vi "Multi-Device Tx Streaming Time (Host).vi"() -> ()   [LabVIEW 2015]
doc: "This template is for the Simple NI-USRP Streaming design, a design that shows the basics of streaming data to and from an NI USRP-294x/295x device. Refer to the block diagram for more information about how to use this template."
uses:
  <vilib>/Utility/error.llb/DialogType.ctl
  <vilib>/userdefined/Silver/nirio_resource_slv.ctl
  SubVIs/Start Trigger.ctl
panel:
  in  "config tab":enum32{"Tx Configuration"}(tab)
  in  "tx config":T2={"rf enable 0"=TRUE, "rf config 0"={"antenna"="TX1", "frequency"=2000000000.0, "lo frequency"=-1.0, "level"=0.0}, "rf enable 1"=TRUE, "rf config 1"={"antenna"="TX1", "frequency"=2000000000.0, "lo frequency"=-1.0, "level"=0.0}, "transfer mode"=enum."Finite", "sample rate"=10000000.0, "number of samples"=8192, "start trigger"=enum."Future Time Event", "tone frequency"=100000.0} {"tone frequency" format="%#.3pHz"; "sample rate" format="%#.3pS/s"; "rf config 0"."level" format="%#_gdBm"; "rf config 0"."lo frequency" format="%#.3pHz"; "rf config 0"."frequency" format="%#.3pHz"; "rf config 1"."level" format="%#_gdBm"; "rf config 1"."lo frequency" format="%#.3pHz"; "rf config 1"."frequency" format="%#.3pHz"}
  in  "tx.stop":bool
  out "generating":bool caption="Generating"
  in  "USRP RIO devices":T3[](array[typedef])=["RIO0", "RIO1"] caption="USRP RIO Devices"
  in  "reference frequency source":string(combo)="REF IN" caption="Reference Frequency Source"
  in  "indicator tab":T4(tab)
  out "tx.waveform":waveform(dbl)[](graph) caption="Output Waveform"
  out "tx.coerced config":T5(array[cluster]) caption="Tx" {"coerced sample rates" format="%#.3pS/s"; "coerced levels" format="%#.3gdBm"; "coerced lo frequencies" format="%#.3pHz"; "coerced frequencies" format="%#.3pHz"}
  # "This template is for the Simple NI-USRP Streaming design, a design that shows the basics of streaming data on an NI 294x/295x device. See the block diagram for more information on how to use this template."
  # "Multi-Device Tx Streaming with Time"
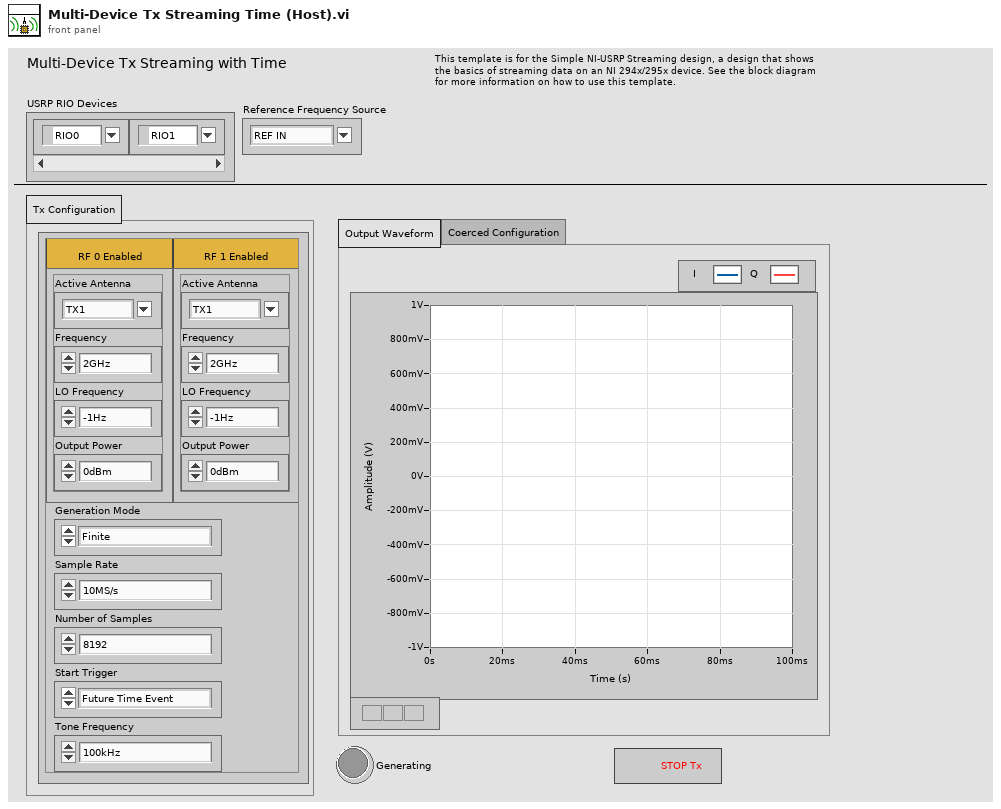
[diagram p1: front panel]
types:
  T1 = typedef "Start Trigger.ctl" = enum8{"Software", "Digital Edge", "Rx Start Trigger", "Tx Start Trigger", "Immediate", "Future Time Event"}
  T2 = cluster{"rf enable 0":bool, "rf config 0":cluster{"antenna":string, "frequency":dbl, "lo frequency":dbl, "level":dbl}, "rf enable 1":bool, "rf config 1":cluster{"antenna":string, "frequency":dbl, "lo frequency":dbl, "level":dbl}, "transfer mode":enum16{"Finite", "Continuous"}, "sample rate":dbl, "number of samples":u32, "start trigger":T1, "tone frequency":dbl}
  T3 = typedef "nirio_resource_slv.ctl" = tag
  T4 = enum32{"Output Waveform", "Coerced Configuration"}
  T5 = cluster{"coerced frequencies":dbl[], "coerced lo frequencies":dbl[], "coerced levels":dbl[], "coerced sample rates":dbl[]}[]
  T6 = typedef "DialogType.ctl" = u16
  T7 = cluster{"tx config":cluster{"rf enable 0":bool, "rf config 0":cluster{"antenna":string, "frequency":dbl, "lo frequency":dbl, "level":dbl}, "rf enable 1":bool, "rf config 1":cluster{"antenna":string, "frequency":dbl, "lo frequency":dbl, "level":dbl}, "transfer mode":enum16{"Finite", "Continuous"}, "sample rate":dbl, "number of samples":u32, "start trigger":T1, "tone frequency":dbl}, "reference frequency source":string, "tx.enabled channels":string[], "I":i16[], "Q":i16[], "tx.coerced configurations":cluster{"coerced frequencies":dbl[], "coerced lo frequencies":dbl[], "coerced levels":dbl[], "coerced sample rates":dbl[]}}
  T8 = typedef "niUsrpRio Config v1 Host.lvlib/niUsrpRio Session.ctl" = cluster{"FPGA Interface":refnum<k20>, "RIO Interface Number":u32, "Data Clock Rate":u32, "FPGA Data Clock Rate":u32, "Global Settings Register Bus":T9, "Radio 0 Settings Register Bus":T9, "Radio 1 Settings Register Bus":T9, "Radio Settings Bus Semaphore":T10, "DB Queues":T11[], "Characterization Data Valid?":bool, "EEPROM Header":T12, "Device Data Header":T13, "EEPROM Characterization Header":T14, "Characterization Data":T15[], "FPGA Current Version":u32, "FPGA Oldest Compatible Version":u32, "Fixed Logic Current Version":u32, "Fixed Logic Oldest Compatible Version":u32, "FPGA Radio Settings Bus Current Version":u32, "FPGA Radio Settings Bus Oldest Compatible Version":u32, "FPGA Board Config Current Version":u32, "FPGA Board Config Oldest Compatible Version":u32, "Daughterboard Clock Rate":u32}
  T9 = typedef "niInstr Register Bus v0 Host.lvlib/Register Bus Session.ctl" = refnum<queue>
  T10 = typedef "Semaphore RefNum" = refnum<k1>
  T11 = typedef "niUsrpRio Config v1 Host.lvlib/DB Queue Reference.ctl" = refnum<queue>
  T12 = typedef "niUsrpRio Config v1 Host.lvlib/EEPROM Header.ctl" = cluster{"Checksum":u32, "Product Code":u16, "Hardware Current Version":u16, "Hardware Oldest Compatible Version":u16, "EEPROM Map Current Version":u16, "EEPROM Map Oldest Compatible Version":u16, "User Password":string, "Pointer to Factory Header":u32, "Pointer to User Header":u32, "Recommended Interval":u16, "Number of Reserved Bytes":i32, "Number of Daughterboards":u8, "Daughterboard IDs":u16[], "Daughterboard Serial Numbers":string[]}
  T13 = typedef "niUsrpRio Config v1 Host.lvlib/EEPROM Device Data Header.ctl" = cluster{"Checksum":u32, "Number of Channels":u8, "Number of Gain Settings":u16[], "Pointer to Characterization Data":u32[], "Number of Reserved Bytes":i32, "Number of Frequencies":u16[]}
  T14 = typedef "niUsrpRio Config v1 Host.lvlib/EEPROM Characterization Header.ctl" = cluster{"Checksum":u32, "Date":timestamp, "Temperature":sgl, "Misc. Info":string, "Pointer to Device Data Header":u32, "Number of Reserved Bytes":i32}
  T15 = typedef "niUsrpRio Config v1 Host.lvlib/Characterization Data.ctl" = cluster{"Gains[dB]":dbl[], "Frequencies [Hz]":dbl[], "IQ Imbalance Table":T16[], "Measured Gains[dB]":dbl[][]}
  T16 = typedef "niUsrpRio Config v1 Host.lvlib/IQ Imbalance.ctl" = cluster{"Gain Imbalance [linear]":dbl, "Phase Imbalance [radians]":dbl, "Offset":cdb}
  T17 = cluster{"coerced frequencies":dbl[], "coerced lo frequencies":dbl[], "coerced levels":dbl[], "coerced sample rates":dbl[]}
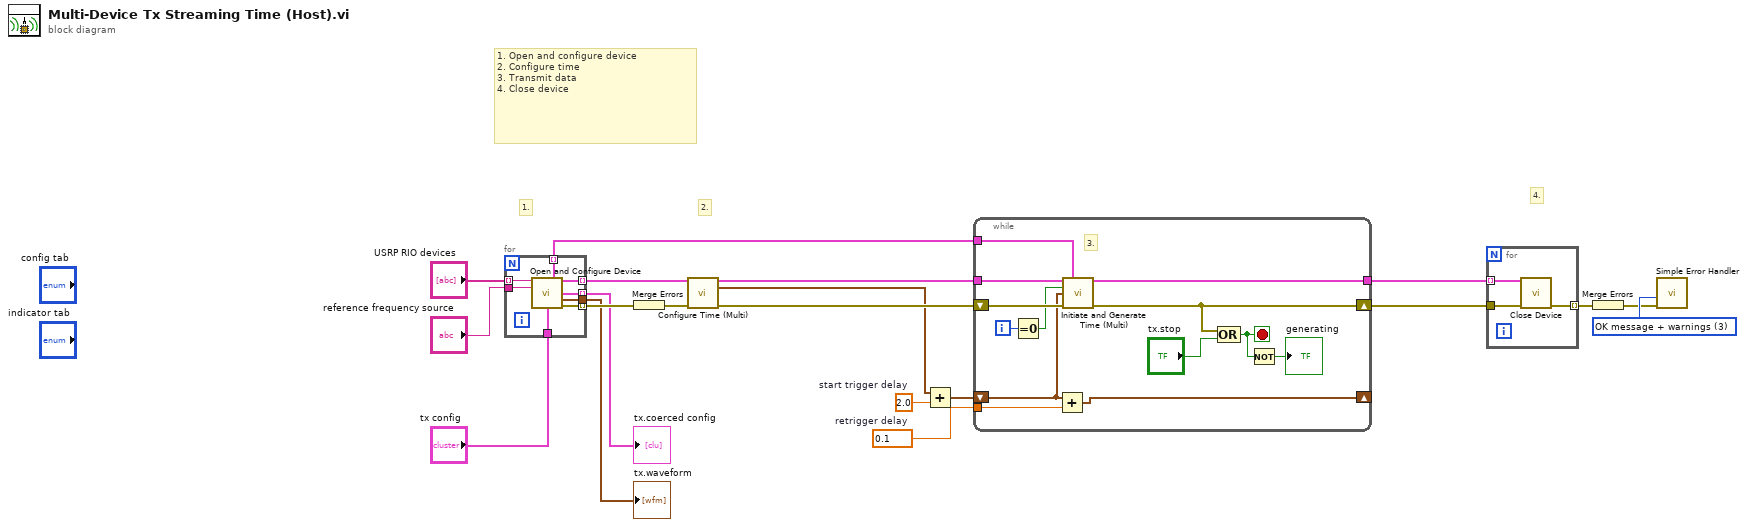
[diagram p0: block diagram]
diagram:
  w4 = 2.0  # start trigger delay
  w3 = 0.1  # retrigger delay
  w17 = T6 3 items=["no dialog", "OK message", "continue or stop message", "OK message + warnings", "continue/stop + warnings"] ("type of dialog (OK msg:1)")
  # "4."
  # "2."
  # "1. Open and configure device\n2. Configure time\n3. Transmit data\n4. Close device"
  # "1."
  n1 = for {
    tunnel: [w28] -> w18 mode=indexing
    tunnel: "tx config" -> [w27]
    tunnel: "reference frequency source" -> [w26]
    tunnel: [w25] -> w7 mode=indexing
    tunnel: [w24] -> w13
    tunnel: [w23] -> w12 mode=indexing
    tunnel: [w22] -> w10 mode=indexing
    tunnel: "USRP RIO devices" -> [w21] mode=indexing
    n2 = call "Open and Configure Device.vi"("USRP RIO Device"=w21, "reference frequency source"=w26, "tx config"=w27) -> ("tx channels"=w22:T7, "niUsrpRio Session (out)"=w23:T8, "tx.coerced configurations"=w25:T17, "tx.output waveform"=w24:waveform(dbl)[], "error out"=w28:errorcluster)  [unwired: 6 in, 2 out]
  }
  "tx.waveform" <- w13
  "tx.coerced config" <- w7
  n3 = Merge Errors(w18) -> (w5:errorcluster)
  n4 = call "Configure Time (Multi).vi"("niUsrpRio Sessions"=w12, "error in"=w5) -> ("niUsrpRio Sessions (out)"=w11:T8[], "time"=w19:timestamp, "error out"=w20:errorcluster)  [unwired: 11 in]
  n5 = Add(x=w19, y=w4) -> (x+y=w2:timestamp)
  n6 = while {
    tunnel: w11 -> [w39]
    tunnel: w10 -> [w34]
    shift-right: [w37] -> w6
    shift-left: w20 -> [w38]
    tunnel: w3 -> [w32]
    shift-right: [w30] -> _
    shift-left: w2 -> [w31]
    tunnel: [w29] -> w1
    i -> [w36]
    stop <- w35 stop-if-true
    # "3."
    # "Acquire and Fetch a waveform"
    n7 = Equal To 0?(x=w36) -> (x = 0?=w33:bool)
    n8 = Add(x=w31, y=w32) -> (x+y=w30:timestamp)
    n9 = call "Initiate and Generate Time (Multi).vi"("niUsrpRio Sessions"=w39, "tx channels"=w34, "first iteration"=w33, "start trigger time"=w31, "error in"=w38) -> ("niUsrpRio Sessions (out)"=w29:T8[], "error out"=w37:errorcluster)  [unwired: 9 in]
    n10 = Compound Arithmetic op=OR(w37, "tx.stop") -> (w35:bool)
    n11 = Not(x=w35) -> (.not. x?=→"generating":bool)
  }
  n12 = for {
    tunnel: w6 -> [w43]
    tunnel: [w44] -> w16 mode=indexing
    tunnel: w1 -> [w42] mode=indexing
    n13 = call "Close Device.vi"("niUsrpRio Session"=w42, "error in"=w43) -> ("error out"=w44:errorcluster)  [unwired: 13 in]
  }
  n14 = Merge Errors(w16) -> (w8:errorcluster)
  n15 = call <vilib>:"Simple Error Handler.vi"("type of dialog (OK msg:1)"=w17, "error in (no error)"=w8) -> ()  [unwired: 3 in, 5 out]
